vi "Benchmark Custom 1.vi"(7 "Reinit":bool, 8 "error in (no error)":errorcluster, 9 "Y":i64, 10 "X":i64, 11 "CIFCorePlugin in":refnum<class "CIFCorePlugin.lvclass">) -> (0 "error out":errorcluster, 3 "CIFCorePlugin out":refnum<class "CIFCorePlugin.lvclass">)   [LabVIEW 2021, in "CIFCorePlugin.lvclass"]
doc: "Load a new data value into the statistics class. The new value will be calculated by subracting the X value from the Y value. This VI is useful for benchmarking where a timestamp is taken before and after a function. The results of this benchmark will automatically be reported through the plugin statistics."
uses:
  CIFCorePlugin.lvclass
  CIFCorePlugin.lvclass/CIFCorePlugin.ctl
  <vilib>/CIF Foundation/CIF Utilities/Statistics/I64/Stats_I64_CIF_U.lvclass/Stats_I64_CIF_U.ctl
  <vilib>/CIF Foundation/CIF Utilities/Statistics/I64/Load X minus Y Delta.vi/dfabcf33-0dbc-4041-80a5-3dc0c86d2989.vi
  <vilib>/CIF Foundation/CIF Utilities/Statistics/I64/Load X minus Y Delta.vi/dfabcf33-0dbc-4041-80a5-3dc0c86d2989.vi/9eb60a9a-770f-4d2d-8b3f-8465c267ecc9.vi
  <vilib>/CIF Foundation/CIF Utilities/Statistics/I64/Stats_I64_CIF_U.lvclass
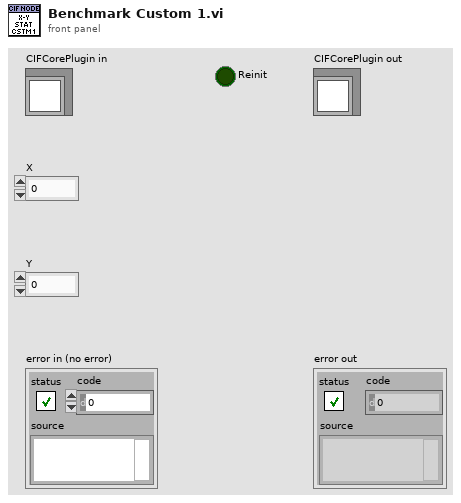
[diagram p1: front panel]
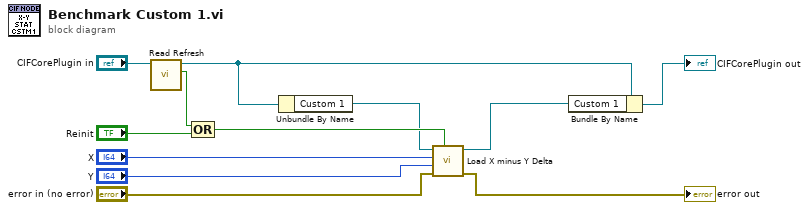
[diagram p0: block diagram]
diagram:
  n1 = call "Read Refresh.vi"("CIFCorePlugin in"="CIFCorePlugin in") -> ("Refresh"=w5:bool, "CIFCorePlugin out"=w3:refnum<class "CIFCorePlugin.lvclass">)  [unwired: 8 in, 1 out]
  n2 = Compound Arithmetic op=OR(w5, "Reinit") -> (w4:bool)
  n3 = Unbundle By Name(w3) -> ("Custom 1"=w2:refnum<class "Stats_I64_CIF_U.lvclass">)
  n4 = call <vilib>:"Load X minus Y Delta.vi"("Reinit"=w4, "error in (no error)"="error in (no error)", "Y"="Y", "X"="X", "Stats_I64_CIF_U in"=w2) -> ("error out"=→"error out":errorcluster, "Stats_I64_CIF_U out"=w1:refnum<class "Stats_I64_CIF_U.lvclass">)  [unwired: 5 in]
  n5 = Bundle By Name(cluster=w3, "Custom 1"=w1) -> (→"CIFCorePlugin out":refnum<class "CIFCorePlugin.lvclass">)
